vi "校准记录.vi"(8 "error in (no error)":errorcluster, 9 "曲线模型":T1={"标液浓度1"=0.0, "测量吸光度1"=0.0, "样品1启用"=FALSE, "标液浓度2"=0.0, "测量吸光度2"=0.0, "样品2启用"=FALSE, "标液浓度3"=0.0, "测量吸光度3"=0.0, "样品3启用"=FALSE, "标液浓度4"=0.0, "测量吸光度4"=0.0, "样品4启用"=FALSE, "标液浓度5"=0.0, "测量吸光度5"=0.0, "样品5启用"=FALSE, "模型"=enum."线性", "精度"=4.0, "XY图"=[], "拟合公式"="", "r^2"=0.0, "标样一校准时间"=timestamp(0 s since 1904-01-01), "标样二校准时间"=timestamp(0 s since 1904-01-01), "标样三校准时间"=timestamp(0 s since 1904-01-01), "标样四校准时间"=timestamp(0 s since 1904-01-01), "标样五校准时间"=timestamp(0 s since 1904-01-01), "二次方程"={"c"=0.0, "x"=0.0, "x^2"=0.0}, "标定时间"=timestamp(0 s since 1904-01-01)} {"标定时间" format="%<%m/%d/%y %H:%M:%S>T"; "标样五校准时间" format="%<%m/%d/%y %H:%M:%S>T"; "标样四校准时间" format="%<%m/%d/%y %H:%M:%S>T"; "标样三校准时间" format="%<%m/%d/%y %H:%M:%S>T"; "标样二校准时间" format="%<%m/%d/%y %H:%M:%S>T"; "标样一校准时间" format="%<%m/%d/%y %H:%M:%S>T"; "r^2" format="%.7f"; "测量吸光度5" format="%#.6f"; "测量吸光度4" format="%#.6f"; "测量吸光度3" format="%#.6f"; "测量吸光度2" format="%#.6f"; "测量吸光度1" format="%#.6f"}, 10 "量程":enum16{"低量程", "高量程"}(ring), 11 "校准参数":u16(ring) items=["总氮"=2, "总磷"=1]) -> (0 "error out":errorcluster)   [LabVIEW 2016, in "斯坦道氨氮.lvlib"]
panel:
  out "结果字符串":string
  # "校准时间"
  # "标液浓度"
  # "吸光值显示"
  # "标液一"
  # "标液二"
  # "标液三"
  # "零点"
  # "跨度"
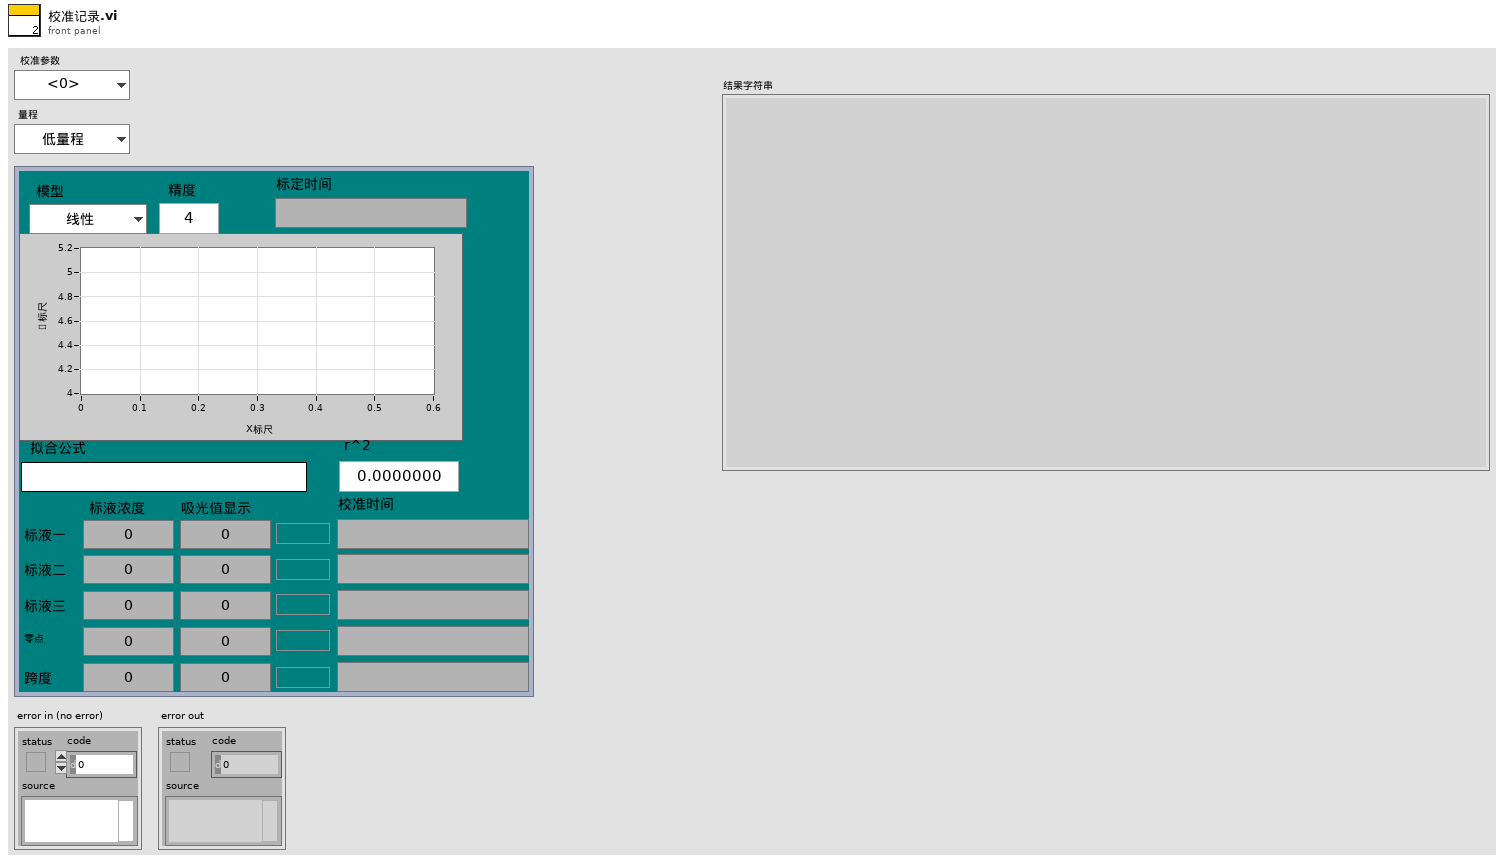
[diagram p1: front panel]
types:
  T1 = cluster{"标液浓度1":dbl, "测量吸光度1":dbl, "样品1启用":bool, "标液浓度2":dbl, "测量吸光度2":dbl, "样品2启用":bool, "标液浓度3":dbl, "测量吸光度3":dbl, "样品3启用":bool, "标液浓度4":dbl, "测量吸光度4":dbl, "样品4启用":bool, "标液浓度5":dbl, "测量吸光度5":dbl, "样品5启用":bool, "模型":enum32{"线性", "多项式"}, "精度":dbl, "XY图":cluster{"X Values":dbl[], "Y Values":dbl[]}[], "拟合公式":string, "r^2":dbl, "标样一校准时间":timestamp, "标样二校准时间":timestamp, "标样三校准时间":timestamp, "标样四校准时间":timestamp, "标样五校准时间":timestamp, "二次方程":cluster{"c":dbl, "x":dbl, "x^2":dbl}, "标定时间":timestamp}
  T2 = typedef "校准日志字段定义.ctl" = cluster{"时间":timestamp, "参数":string, "日志信息":string, "流程参数":string}
  T3 = typedef "数据库类型.ctl" = enum16{"Access", "SQLite"}
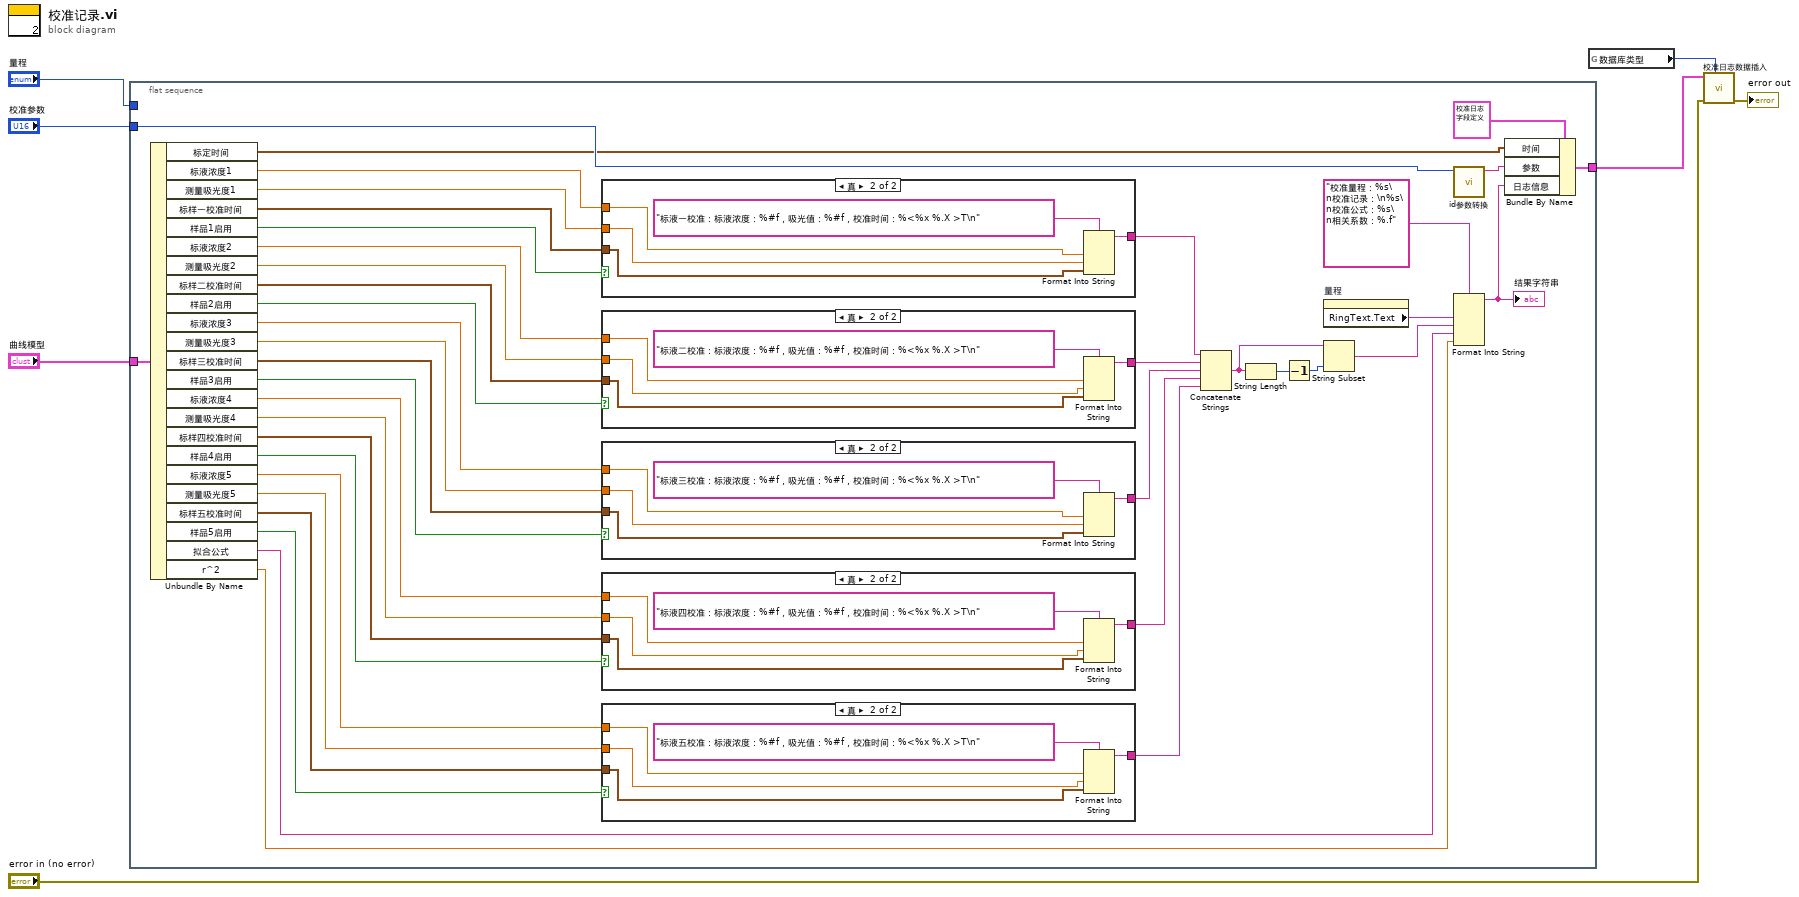
[diagram p0: block diagram]
diagram:
  n1 = flat-sequence {
    tunnel: "校准参数" -> [w47]
    tunnel: "量程" -> [_]
    tunnel: "曲线模型" -> [w42]
    tunnel: [w45] -> w3
    frame #0 {
      n2 = Unbundle By Name(w42) -> ("标定时间"=w10:timestamp, "标液浓度1"=w40:dbl, "测量吸光度1"=w39:dbl, "标样一校准时间"=w38:timestamp, "样品1启用"=w41:bool, "标液浓度2"=w37:dbl, "测量吸光度2"=w36:dbl, "标样二校准时间"=w35:timestamp, "样品2启用"=w34:bool, "标液浓度3"=w33:dbl, "测量吸光度3"=w32:dbl, "标样三校准时间"=w31:timestamp, "样品3启用"=w30:bool, "标液浓度4"=w29:dbl, "测量吸光度4"=w28:dbl, "标样四校准时间"=w27:timestamp, "样品4启用"=w26:bool, "标液浓度5"=w25:dbl, "测量吸光度5"=w24:dbl, "标样五校准时间"=w23:timestamp, "样品5启用"=w22:bool, "拟合公式"=w16:string, "r^2"=w15:dbl)
      n3 = case shown="真" w41 {
        tunnel: w40 -> [_ w71]
        tunnel: w39 -> [_ w70]
        tunnel: w38 -> [_ w69]
        tunnel: [_ w68] -> w21
        frame False {
        }
        frame True {
          n4 = Format Into String(format string="标液一校准：标液浓度：%#f，吸光值：%#f，校准时间：%<%x %.X >T\n" ("格式字符串"), w71, w70, w69) -> (resulting string=w68:string)  [unwired: 2 in, 1 out]
        }
      }
      n5 = case shown="真" w34 {
        tunnel: w37 -> [_ w66]
        tunnel: w36 -> [_ w65]
        tunnel: w35 -> [_ w64]
        tunnel: [_ w63] -> w20
        frame False {
        }
        frame True {
          n6 = Format Into String(format string="标液二校准：标液浓度：%#f，吸光值：%#f，校准时间：%<%x %.X >T\n" ("格式字符串"), w66, w65, w64) -> (resulting string=w63:string)  [unwired: 2 in, 1 out]
        }
      }
      n7 = case shown="真" w30 {
        tunnel: w33 -> [_ w61]
        tunnel: w32 -> [_ w60]
        tunnel: w31 -> [_ w59]
        tunnel: [_ w58] -> w19
        frame False {
        }
        frame True {
          n8 = Format Into String(format string="标液三校准：标液浓度：%#f，吸光值：%#f，校准时间：%<%x %.X >T\n" ("格式字符串"), w61, w60, w59) -> (resulting string=w58:string)  [unwired: 2 in, 1 out]
        }
      }
      n9 = case shown="真" w26 {
        tunnel: w29 -> [_ w56]
        tunnel: w28 -> [_ w55]
        tunnel: w27 -> [_ w54]
        tunnel: [_ w53] -> w18
        frame False {
        }
        frame True {
          n10 = Format Into String(format string="标液四校准：标液浓度：%#f，吸光值：%#f，校准时间：%<%x %.X >T\n" ("格式字符串"), w56, w55, w54) -> (resulting string=w53:string)  [unwired: 2 in, 1 out]
        }
      }
      n11 = case shown="真" w22 {
        tunnel: w25 -> [_ w51]
        tunnel: w24 -> [_ w50]
        tunnel: w23 -> [_ w49]
        tunnel: [_ w48] -> w17
        frame False {
        }
        frame True {
          n12 = Format Into String(format string="标液五校准：标液浓度：%#f，吸光值：%#f，校准时间：%<%x %.X >T\n" ("格式字符串"), w51, w50, w49) -> (resulting string=w48:string)  [unwired: 2 in, 1 out]
        }
      }
      n13 = Concatenate Strings(w21, w20, w19, w18, w17) -> (w13:string)
      n14 = String Length(string=w13) -> (length=w12:i32)
      n15 = Decrement(x=w12) -> (x-1=w11:i32)
      n16 = property on="量程" class="Enum (严格)"() -> ("RingText.Text"=w9:string)  [unwired: 2 in, 2 out]
      n17 = String Subset(string=w13, length (rest)=w11) -> (substring=w14:string)  [unwired: 1 in]
      n18 = call "id参数转换.vi"("id"=w47) -> ("table输出"=w46:string)  [unwired: 9 in, 1 out]
      n19 = Format Into String(format string="校准量程：%s\n校准记录：\n%s\n校准公式：%s\n相关系数：%.f" ("格式字符串"), w9, w14, w16, w15) -> (resulting string=w44:string)  [unwired: 2 in, 1 out]
      "结果字符串" <- w44
      n20 = Bundle By Name(cluster=T2 {"时间"=timestamp(0 s since 1904-01-01), "参数"="", "日志信息"="", "流程参数"=""} ("data"), "时间"=w10, "参数"=w46, "日志信息"=w44) -> (w45:T2)
    }
  }
  n21 = global read "总磷总氮断电保存全局变量.vi" "数据库类型"() -> (w4:T3)
  n22 = call "校准日志数据插入.vi"("data"=w3, "错误输入（无错误）"="error in (no error)", "数据库类型"=w4) -> ("错误输出"=→"error out":errorcluster)  [unwired: 7 in]
